vi "VCL_2_TSV_2_LV_BATCH.vi"(8 "error in (no error)":errorcluster, 11 "path to logfile directory":path=path "C:/Users/Patrick/Desktop/VCL/logfiles") -> (0 "error out":errorcluster)   [LabVIEW 2016, in "VCL_2_DSC.lvclass"]
uses:
  VCL_2_DSC.lvclass
panel:
  out "All txt Files in Dir":path[](array[path])
  out "standard output":string
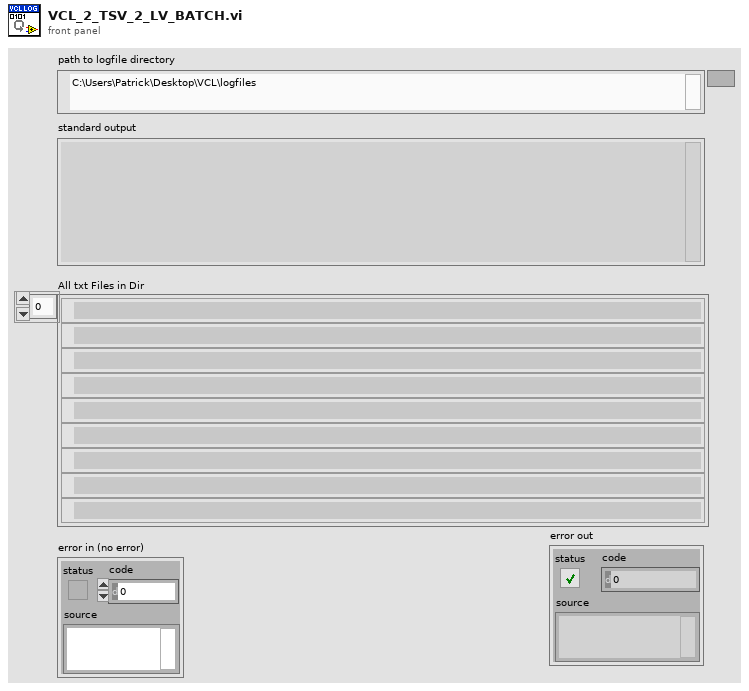
[diagram p1: front panel]
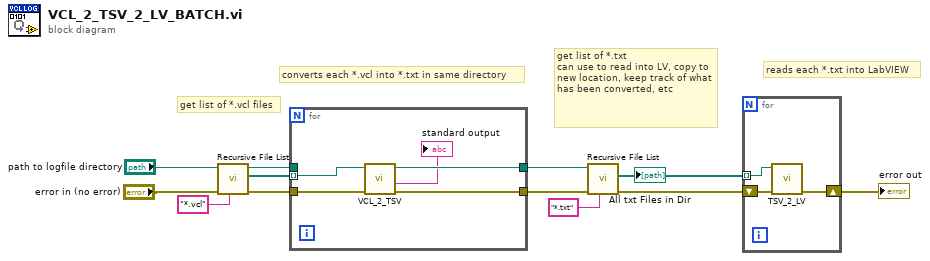
[diagram p0: block diagram]
diagram:
  # "get list of *.txt\ncan use to read into LV, copy to new location, keep track of what has been converted, etc"
  # "reads each *.txt into LabVIEW"
  # "converts each *.vcl into *.txt in same directory"
  # "get list of *.vcl files"
  n1 = call <vilib>:"Recursive File List.vi"("pattern"="*.vcl", "error in (no error)"="error in (no error)", "Folder Path"="path to logfile directory") -> ("error out"=w11:errorcluster, "All Files in Dir"=w10:path[], "dup Folder Path"=w6:path)  [unwired: 4 in, 2 out]
  n2 = for {
    tunnel: w11 -> [w16]
    tunnel: w10 -> [w13] mode=indexing
    tunnel: [w17] -> w7
    tunnel: w6 -> [_]
    tunnel: [w15] -> w5
    n3 = call "VCL_2_TSV.vi"("error in (no error)"=w16, "Path to VCL file"=w13) -> ("error out"=w17:errorcluster, "standard output"=→"standard output":string, "path to logfile directory"=w15:path)  [unwired: 6 in, 1 out]
  }
  n4 = call <vilib>:"Recursive File List.vi"("pattern"="*.txt", "error in (no error)"=w7, "Folder Path"=w5) -> ("error out"=w4:errorcluster, "All Files in Dir"=w2:path[])  [unwired: 4 in, 3 out]
  "All txt Files in Dir" <- w2
  n5 = for {
    shift-right: [w19] -> w3
    shift-left: w4 -> [w20]
    tunnel: w2 -> [w18] mode=indexing
    n6 = call "TSV_2_LV.vi"("error in (no error)"=w20, "file path (dialog if empty)"=w18) -> ("error out"=w19:errorcluster)  [unwired: 9 in]
  }
  "error out" <- w3
